vi "Untitled 4.vi"(7 "Sheet Name":string, 8 "error in":errorcluster, 9 "Values":variant[](array[variant]), 10 "Cell Address":string, 11 "SpreadsheetDocument":refnum<k24>) -> (0 "error out":errorcluster, 3 "SpreadsheetDocument out":refnum<k24>)   [LabVIEW 2021, in "Open Xml.lvlib"]
uses:
  Source/Open Xml.lvlib
  D:/git/Open-Xml-LabVIEW/dll/DocumentFormat.OpenXml.dll
  dll/DocumentFormat.OpenXml.dll
  <vilib>/Utility/Data Type/NI_Data Type.lvlib
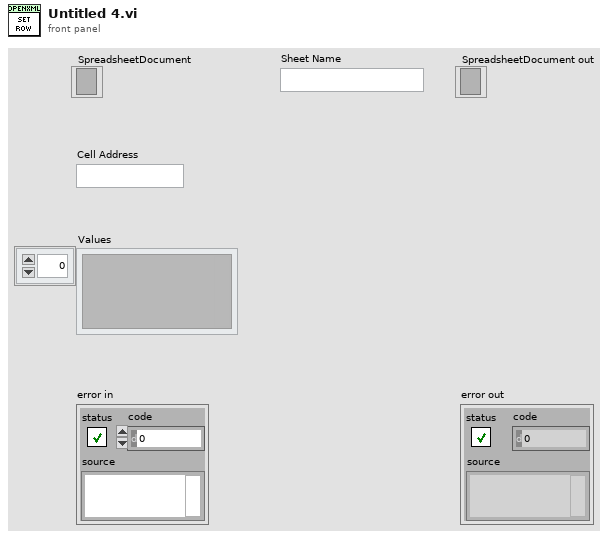
[diagram p1: front panel]
types:
  T1 = typedef "NI_Data Type.lvlib/Data Type.ctl" = enum8{"Invalid Type", "Void", "I8", "I16", "I32", "I64", "U8", "U16", "U32", "U64", "Single Float", "Double Float", "Extended Float", "Single Complex", "Double Complex", "Extended Complex", "Enum U8", "Enum U16", "Enum U32", "Enum U64", "Single Float With Unit", "Double Float With Unit", "Extended Float With Unit", "Single Complex with Unit", "Double Complex with Unit", "Extended Complex with Unit", "Boolean", "String", "Path", "Picture", "Tag", "Array", "Cluster", "Variant", "LV Variant", "Waveform", "Timestamp", "Digital Waveform", "Digital Data", "ExpressData", "Refnum", "External Data", "VI", "Poly VI", "LabVIEW Class Instance", "Fixed Point", "Set Collection", "Map Collection"}
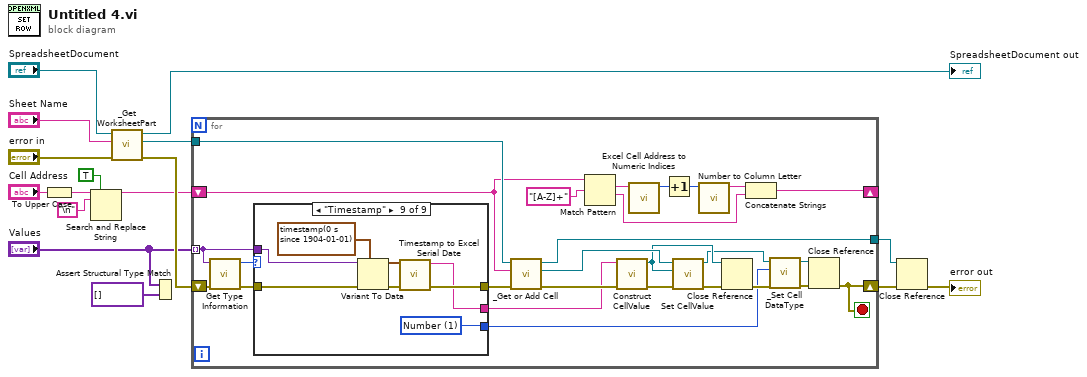
[diagram p0: block diagram]
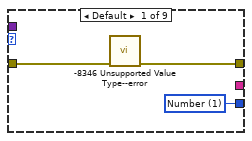
[diagram p2: hidden frame]
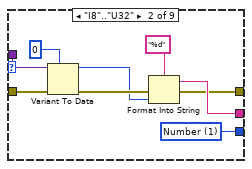
[diagram p3: hidden frame]
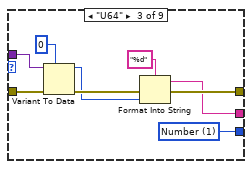
[diagram p4: hidden frame]
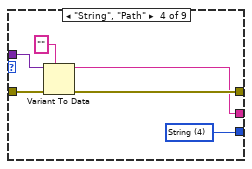
[diagram p5: hidden frame]
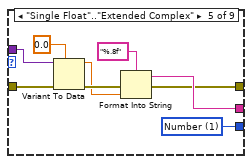
[diagram p6: hidden frame]
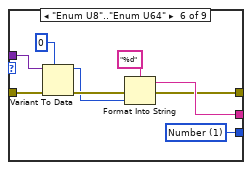
[diagram p7: hidden frame]
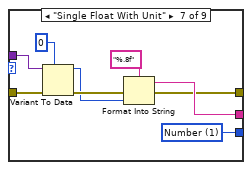
[diagram p8: hidden frame]
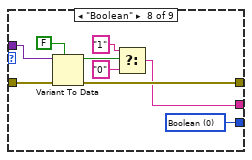
[diagram p9: hidden frame]
diagram:
  n1 = To Upper Case(1:"Cell Address") -> (0:w4:string)
  n2 = Search and Replace String(replace all?=TRUE ("replace all? (F)"), input string=w4, search string="\n") -> (result string=w6:string)  [unwired: 5 in, 3 out]
  n3 = call "_Get WorksheetPart.vi"("error in"="error in", "Sheet Name"="Sheet Name", "SpreadsheetDocument in"="SpreadsheetDocument") -> ("error out"=w14:errorcluster, "WorksheetPart"=w13:refnum<k24>, "SpreadsheetDocument out"=→"SpreadsheetDocument out":refnum<k24>)  [unwired: 6 in]
  n4 = Assert Structural Type Match(0:variant[] [], 1:"Values") -> ()
  n5 = for {
    tunnel: "Values" -> [w41] mode=indexing
    shift-right: [w18] -> w2
    shift-left: w14 -> [w43]
    shift-right: [w32] -> _
    shift-left: w6 -> [w21]
    tunnel: w13 -> [w31]
    tunnel: [w17] -> w1
    stop <- w18 stop-if-true
    n6 = call <vilib>:"Get Type Information.vi"("error in (no error)"=w43, "variant"=w41) -> ("error out"=w42:errorcluster, "type"=w39:T1)  [unwired: 5 in, 3 out]
    n7 = case shown="\"Timestamp\"" w39 {
      tunnel: w42 -> [w46 w55 w64 w70 w79 w88 w97 w106 w113]
      tunnel: w41 -> [_ w51 w62 w68 w74 w83 w92 w105 w111]
      tunnel: [_ w53 w57 w66 w77 w86 w95 w99 w108] -> w28
      tunnel: [w45 w48 w60 w67 w76 w85 w94 w103 w112] -> w40
      tunnel: [w44 w47 w56 w65 w71 w80 w90 w98 w107] -> w19
      frame Default {
        w44 = 1 items=["Boolean", "Number", "Error", "SharedString", "String", "InlineString", "Date"] ("Datatype")
        n8 = call "-8346 Unsupported Value Type--error.vi"("error in"=w46) -> ("error out"=w45:errorcluster)  [unwired: 10 in]
      }
      frame "I8".."U32" {
        w47 = 1 items=["Boolean", "Number", "Error", "SharedString", "String", "InlineString", "Date"] ("Datatype")
        n9 = Variant To Data(error in=w55, type=i64 0, Variant=w51) -> (data=w49:i64, error out=w52:errorcluster)
        n10 = Format Into String(format string="%d", error in=w52, w49) -> (resulting string=w53:string, error out=w48:errorcluster)  [unwired: 1 in]
      }
      frame "U64" {
        w56 = 1 items=["Boolean", "Number", "Error", "SharedString", "String", "InlineString", "Date"] ("Datatype")
        n11 = Variant To Data(error in=w64, type=u64 0, Variant=w62) -> (data=w59:u64, error out=w61:errorcluster)
        n12 = Format Into String(format string="%d", error in=w61, w59) -> (resulting string=w57:string, error out=w60:errorcluster)  [unwired: 1 in]
      }
      frame "String", "Path" {
        w65 = 4 items=["Boolean", "Number", "Error", "SharedString", "String", "InlineString", "Date"] ("Datatype")
        n13 = Variant To Data(error in=w70, type="", Variant=w68) -> (data=w66:string, error out=w67:errorcluster)
      }
      frame "Single Float".."Extended Complex" {
        w71 = 1 items=["Boolean", "Number", "Error", "SharedString", "String", "InlineString", "Date"] ("Datatype")
        n14 = Variant To Data(error in=w79, type=0.0, Variant=w74) -> (data=w72:dbl, error out=w75:errorcluster)
        n15 = Format Into String(format string="%.8f", error in=w75, w72) -> (resulting string=w77:string, error out=w76:errorcluster)  [unwired: 1 in]
      }
      frame "Enum U8".."Enum U64" {
        w80 = 1 items=["Boolean", "Number", "Error", "SharedString", "String", "InlineString", "Date"] ("Datatype")
        n16 = Variant To Data(error in=w88, type=u64 0, Variant=w83) -> (data=w81:u64, error out=w84:errorcluster)
        n17 = Format Into String(format string="%d", error in=w84, w81) -> (resulting string=w86:string, error out=w85:errorcluster)  [unwired: 1 in]
      }
      frame "Single Float With Unit" {
        w90 = 1 items=["Boolean", "Number", "Error", "SharedString", "String", "InlineString", "Date"] ("Datatype")
        n18 = Variant To Data(error in=w97, type=u64 0, Variant=w92) -> (data=w89:u64, error out=w93:errorcluster)
        n19 = Format Into String(format string="%.8f", error in=w93, w89) -> (resulting string=w95:string, error out=w94:errorcluster)  [unwired: 1 in]
      }
      frame "Boolean" {
        w98 = 0 items=["Boolean", "Number", "Error", "SharedString", "String", "InlineString", "Date"] ("Datatype")
        n20 = Variant To Data(error in=w106, type=FALSE, Variant=w105) -> (data=w102:bool, error out=w103:errorcluster)
        n21 = Select(t="1", s=w102, f="0") -> (s? t:f=w99:string)
      }
      frame "Timestamp" {
        w107 = 1 items=["Boolean", "Number", "Error", "SharedString", "String", "InlineString", "Date"] ("Datatype")
        n22 = Variant To Data(error in=w113, type=timestamp(0 s since 1904-01-01), Variant=w111) -> (data=w110:timestamp, error out=w112:errorcluster)
        n23 = call "Timestamp to Excel Serial Date.vi"("Timestamp"=w110) -> ("Excel Serial Date"=w108:string)  [unwired: 10 in]
      }
    }
    n24 = call "_Get or Add Cell.vi"("error in"=w40, "Cell Address"=w21, "Worksheetpart in"=w31) -> ("error out"=w30:errorcluster, "Cell"=w26:refnum<k24>, "WorksheetPart out"=w17:refnum<k24>)  [unwired: 6 in]
    n25 = Match Pattern(string=w21, regular expression="[A-Z]+") -> (match substring=w37:string, after substring=w34:string)  [unwired: 1 in, 2 out]
    n26 = call "Construct CellValue.vi"("error in"=w30, "Text"=w28) -> ("error out"=w29:errorcluster, "CellValue out"=w25:refnum<k24>)  [unwired: 8 in]
    n27 = call "Excel Cell Address to Numeric Indices.vi"("Cell Name"=w37) -> ("Column Number"=w36:u32)  [unwired: 9 in, 1 out]
    n28 = Increment(x=w36) -> (x+1=w35:u32)
    n29 = call "Set CellValue.vi"("error in"=w29, "CellValue in"=w25, "Cell in"=w26) -> ("error out"=w27:errorcluster, "Cell out"=w22:refnum<k24>)  [unwired: 7 in]
    n30 = call "Number to Column Letter.vi"("Number"=w35) -> ("Letter"=w33:string)  [unwired: 10 in]
    n31 = Close Reference(reference=w25, error in (no error)=w27) -> (error out=w24:errorcluster)
    n32 = Concatenate Strings(w33, w34) -> (w32:string)
    n33 = call "_Set Cell DataType.vi"("error in"=w24, "Datatype"=w19, "Cell in"=w22) -> ("error out"=w23:errorcluster, "Cell out"=w20:refnum<k24>)  [unwired: 7 in]
    n34 = Close Reference(reference=w20, error in (no error)=w23) -> (error out=w18:errorcluster)
  }
  n35 = Close Reference(reference=w1, error in (no error)=w2) -> (error out=→"error out":errorcluster)
